vi "Set Profile.vi"(7 "Profile Info":T1 {"dt" format="%<%H:%M:%S>t"; "Duration" format="%<%H:%M:%S>t"}, 8 "Error In":errorcluster) -> (0 "Error Out":errorcluster, 1 "Infinite?":bool=TRUE, 2 "dT":dbl, 3 "Waveform Graph":waveform(dbl)(graph)={"t0"=timestamp(0 s since 1904-01-01), "dt"=300.0, "Y"=[-11.666666666666666, -11.666666666666666, -11.666666666666666, -11.666666666666666, -11.666666666666666, -11.666666666666666, -11.666666666666666, -11.666666666666666, -11.666666666666666, -11.666666666666666, -11.666666666666666, -11.666666666666666]})   [LabVIEW 2019, in "GUI.lvlib"]
uses:
  GUI.lvlib
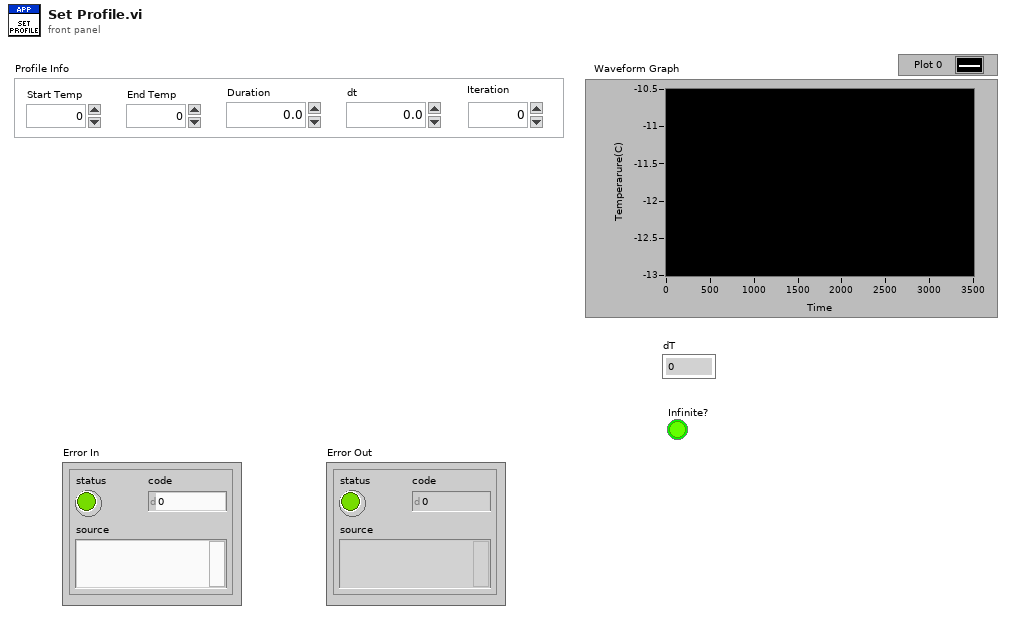
[diagram p1: front panel]
types:
  T1 = cluster{"Start Temp":dbl, "End Temp":dbl, "Duration":dbl, "dt":dbl, "Iteration":i32}
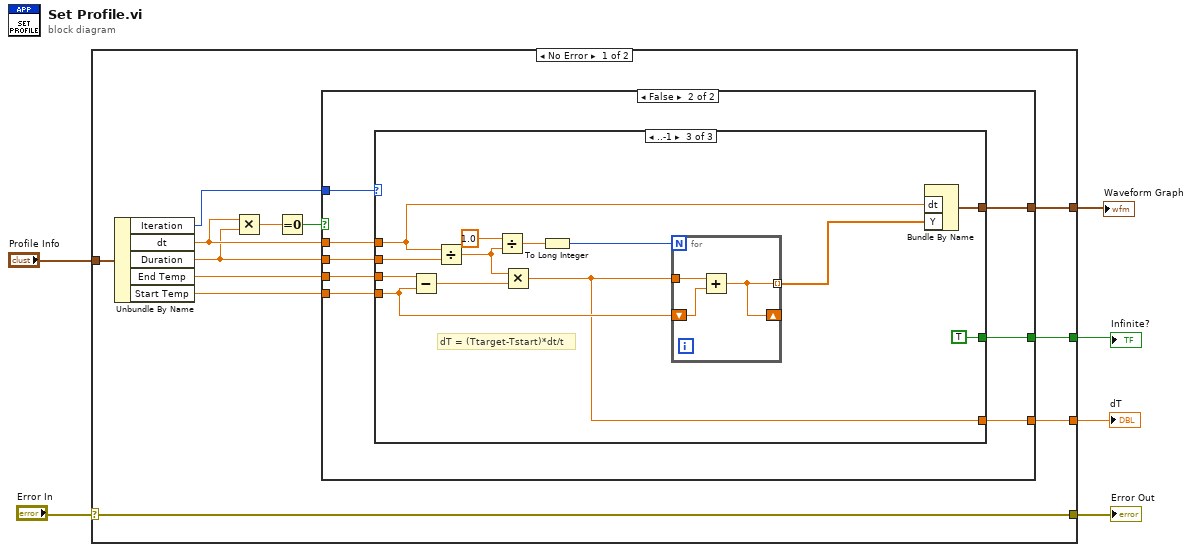
[diagram p0: block diagram]
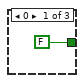
[diagram p3: hidden frame]
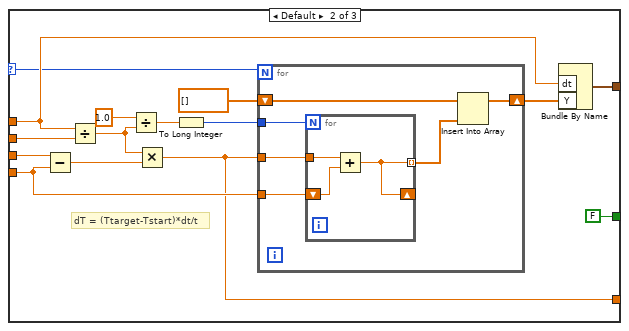
[diagram p4: hidden frame]
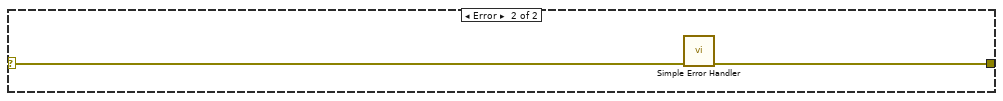
[diagram p5: hidden frame]
diagram:
  n1 = case shown="No Error" "Error In" {
    selector: "Error In" -> [w18 w69]
    tunnel: [w18 w68] -> w5
    tunnel: "Profile Info" -> [w17 _]
    tunnel: [w16 _] -> w4
    tunnel: [w13 _] -> w3
    tunnel: [w7 _] -> w1
    frame No Error {
      n2 = Unbundle By Name(w17) -> ("Iteration"=w8:i32, "dt"=w10:dbl, "Duration"=w9:dbl, "End Temp"=w15:dbl, "Start Temp"=w14:dbl)
      n3 = Multiply(x=w10, y=w9) -> (x*y=w12:dbl)
      n4 = Equal To 0?(x=w12) -> (x = 0?=w11:bool)
      n5 = case shown="False" w11 {
        tunnel: [_ w26] -> w16
        tunnel: w15 -> [_ w25]
        tunnel: w10 -> [_ w24]
        tunnel: w14 -> [_ w23]
        tunnel: [_ w22] -> w13
        tunnel: w9 -> [_ w21]
        tunnel: w8 -> [_ w20]
        tunnel: [_ w19] -> w7
        frame True {
        }
        frame False {
          n6 = case shown="..-1" w20 {
            selector: w20 -> [_ w31 _]
            tunnel: [_ w42 w64] -> w26
            tunnel: w25 -> [_ w41 w63]
            tunnel: w24 -> [_ w35 w57]
            tunnel: w23 -> [_ w34 w56]
            tunnel: [_ w33 w55] -> w22
            tunnel: w21 -> [_ w32 w54]
            tunnel: [FALSE ("Infinite?") FALSE ("Infinite?") TRUE ("Infinite?")] -> w19
            frame 0 {
            }
            frame Default {
              # "dT = (Ttarget-Tstart)*dt/t"
              n7 = Subtract(x=w41, y=w34) -> (x-y=w40:dbl)
              n8 = Divide(x=w35, y=w32) -> (x/y=w39:dbl)
              n9 = Divide(x=1.0 ("dt"), y=w39) -> (x/y=w37:dbl)
              n10 = Multiply(x=w39, y=w40) -> (x*y=w33:dbl)
              n11 = To Long Integer(number=w37) -> (32bit integer=w36:i32)
              n12 = for {
                N: w31 -> [_]
                tunnel: w36 -> [w48]
                tunnel: w34 -> [w47]
                tunnel: w33 -> [w46]
                shift-right: [w44] -> w29
                shift-left: dbl[] [] -> [w43]
                n13 = for {
                  N: w48 -> [_]
                  tunnel: w46 -> [w50]
                  shift-right: [w51] -> _
                  shift-left: w47 -> [w49]
                  tunnel: [w51] -> w45 mode=indexing
                  n14 = Add(x=w50, y=w49) -> (x+y=w51:dbl)
                }
                n15 = Insert Into Array(array=w43, new element=w45) -> (w44:dbl[])  [unwired: 1 in]
              }
              n16 = Bundle By Name("dt"=w35, "Y"=w29) -> (w42:waveform(dbl))  [unwired: 1 in]
            }
            frame ..-1 {
              # "dT = (Ttarget-Tstart)*dt/t"
              n17 = Subtract(x=w63, y=w56) -> (x-y=w62:dbl)
              n18 = Divide(x=w57, y=w54) -> (x/y=w61:dbl)
              n19 = Divide(x=1.0 ("dt"), y=w61) -> (x/y=w59:dbl)
              n20 = Multiply(x=w61, y=w62) -> (x*y=w55:dbl)
              n21 = To Long Integer(number=w59) -> (32bit integer=w58:i32)
              n22 = for {
                N: w58 -> [_]
                tunnel: w55 -> [w66]
                shift-right: [w67] -> _
                shift-left: w56 -> [w65]
                tunnel: [w67] -> w52 mode=indexing
                n23 = Add(x=w66, y=w65) -> (x+y=w67:dbl)
              }
              n24 = Bundle By Name("dt"=w57, "Y"=w52) -> (w64:waveform(dbl))  [unwired: 1 in]
            }
          }
        }
      }
    }
    frame Error {
      n25 = call <vilib>:"Simple Error Handler.vi"("error in (no error)"=w69) -> ("error out"=w68:errorcluster)  [unwired: 4 in, 4 out]
    }
  }
  "Error Out" <- w5
  "Waveform Graph" <- w4
  "dT" <- w3
  "Infinite?" <- w1
